vi "Assert Number of Calls.vi"(8 "error in":errorcluster, 9 "name of call":string, 10 "actual calls":u32, 11 "expected calls":u32) -> (0 "error out":errorcluster, 2 "result":string, 3 "pass":bool)   [LabVIEW 2020, in "MeasurementServerTests.lvlib"]
uses:
  MeasurementServerTests.lvlib
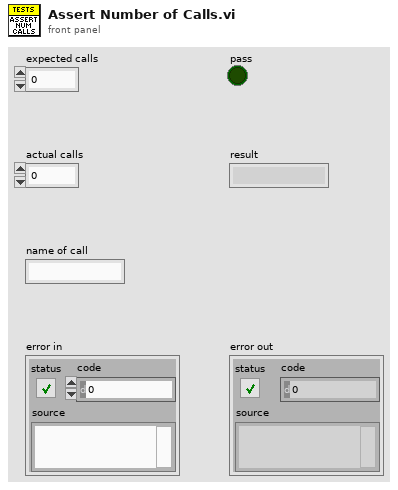
[diagram p1: front panel]
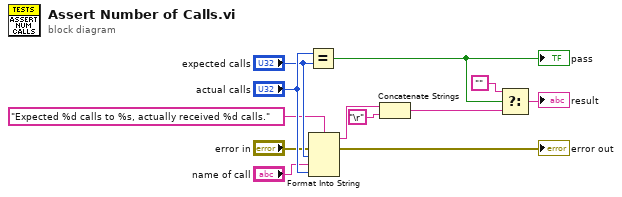
[diagram p0: block diagram]
diagram:
  n1 = Equal?(x="actual calls", y="expected calls") -> (x = y?=w5:bool)
  "pass" <- w5
  n2 = Format Into String(format string="Expected %d calls to %s, actually received %d calls.", error in="error in", "expected calls", "name of call", "actual calls") -> (resulting string=w10:string, error out=→"error out":errorcluster)  [unwired: 1 in]
  n3 = Concatenate Strings(w10, "\r") -> (w12:string)
  n4 = Select(t="", s=w5, f=w12) -> (s? t:f=→"result":string)
